vi "PH_4_Pos_Selector.contents.vi"   [LabVIEW 2014, in "PH_4_Pos_Selector.lvlib"]
doc: "This class is forseen to control up to two Sixpack Axes (class: PH_Sixpack).\n\nThis class is part of the PHELIX user layer."
uses:
  PH_4_Pos_Selector.lvlib
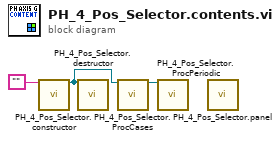
[diagram p0: block diagram]
diagram:
  n1 = call "PH_4_Pos_Selector.constructor.vi"("name"="") -> ("i ref out"=w1:refnum<vi>)  [unwired: 16 in, 2 out]
  n2 = call "PH_4_Pos_Selector.destructor.vi"("i ref in"=w1) -> ()  [unwired: 18 in, 1 out]
  n3 = call "PH_4_Pos_Selector.ProcCases.vi"("i ref in"=w1) -> ("i ref out"=w3:refnum<vi>)  [unwired: 16 in, 2 out]
  n4 = call "PH_4_Pos_Selector.ProcPeriodic.vi"("i ref in"=w3) -> ()  [unwired: 16 in, 3 out]
  n5 = call "PH_4_Pos_Selector.panel.vi"() -> ()  [unwired: 19 in, 1 out]
